vi "MRC Smart IO Set Pwm Output Period.vi"(8 "error in (no error)":errorcluster, 10 "period":enum16{"20ms", "10ms", "5ms", "2ms"}(ring), 11 "deviceIndex":i32) -> (0 "error out":errorcluster)   [LabVIEW 2026, in "MrcLib.lvlib"]
doc: "MRC_Status MRC_CALLCONV MRC_SmartIO_SetPwmOutputPeriod(int32_t deviceIndex,\n MRC_PwmOutputPeriod period);"
uses:
  MrcLib.lvlib
  MrcLib.so
panel:
  # "MRC_PwmOutputPeriod_20ms = 0,\n    MRC_PwmOutputPeriod_10ms,\n    MRC_PwmOutputPeriod_5ms,\n    MRC_PwmOutputPeriod_2ms,"
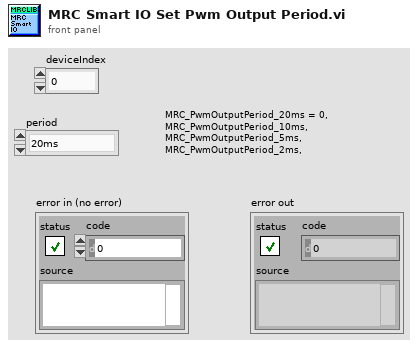
[diagram p1: front panel]
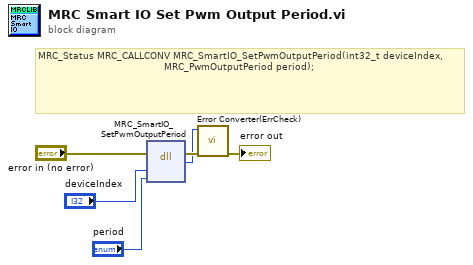
[diagram p0: block diagram]
diagram:
  # "MRC_Status MRC_CALLCONV MRC_SmartIO_SetPwmOutputPeriod(int32_t deviceIndex,\n                                          MRC_PwmOutputPeriod period);"
  n1 = dll-call lib="MrcLib.*" fn="MRC_SmartIO_SetPwmOutputPeriod"(error in="error in (no error)", "deviceIndex"="deviceIndex", "period"="period") -> (error out=w3:errorcluster, w1:i32)  [unwired: 4 in, 1 out]
  n2 = call "Error Converter(ErrCheck).vi"("error in (no error)"=w3, "status"=w1) -> ("error out"=→"error out":errorcluster)  [unwired: 9 in]
